vi "Generate intial guess.vi"(2 "数组":dbl[][](array[numeric])) -> (14 "peak":dbl, 15 "xc":dbl, 16 "yc":dbl, 17 "sigx":i32, 18 "sigy":i32)   [LabVIEW 2013]
panel:
  out "数组 3":ext[](array[numeric])
  out "数组 2":dbl[](array[numeric])
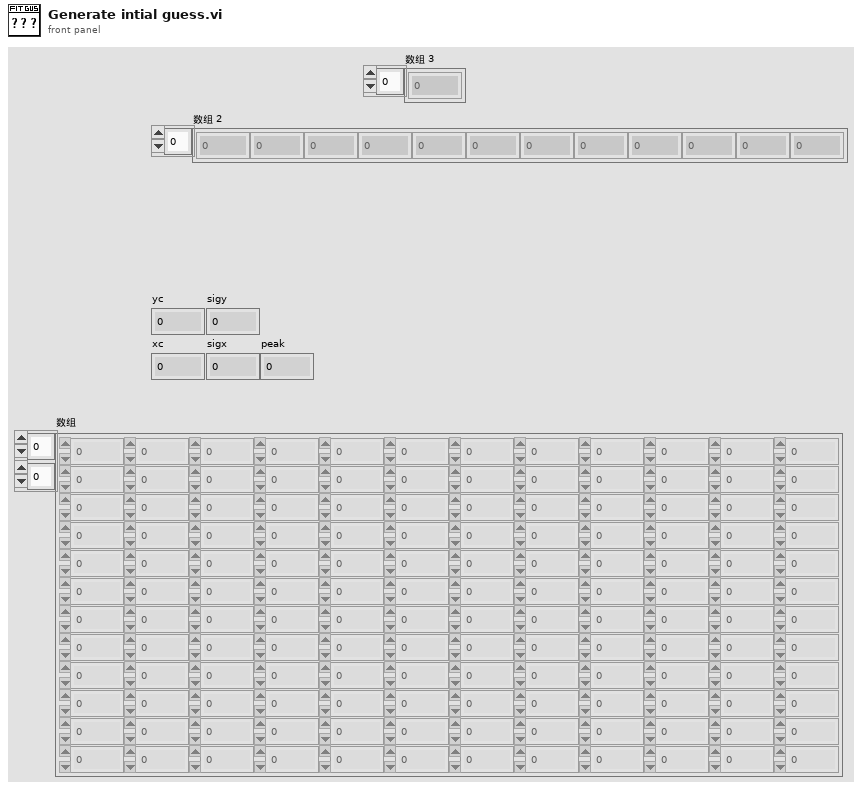
[diagram p1: front panel]
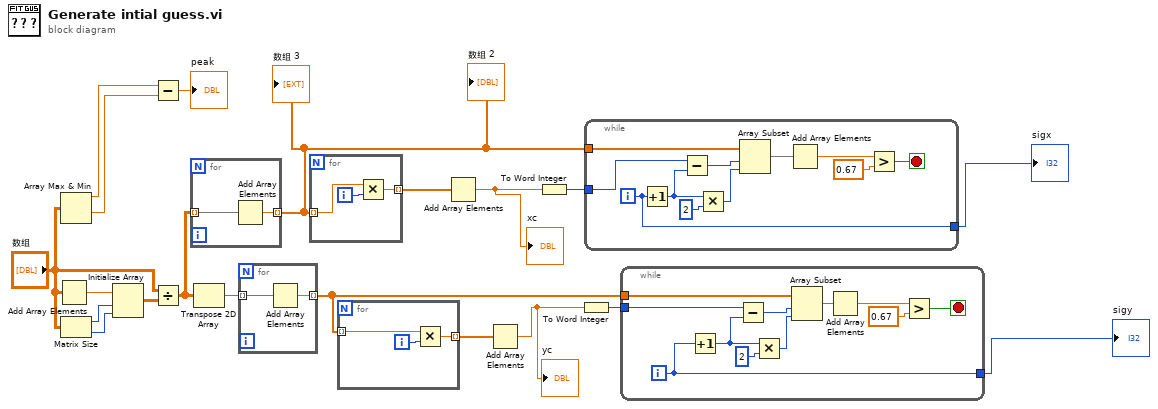
[diagram p0: block diagram]
diagram:
  n1 = Add Array Elements(numeric array="数组") -> (sum=w18:dbl)
  n2 = Array Max & Min(array="数组") -> (max value=w7:dbl, min value=w6:dbl)  [unwired: 2 out]
  n3 = Matrix Size(0:"数组") -> (1:w20:i32, 2:w19:i32)
  n4 = Initialize Array(w18, w20, w19) -> (w17:dbl[][])
  n5 = Subtract(x=w7, y=w6) -> (x-y=→"peak":dbl)
  n6 = Divide(x="数组", y=w17) -> (x/y=w16:dbl[][])
  n7 = for {
    tunnel: w16 -> [w22] mode=indexing
    tunnel: [w21] -> w10 mode=indexing
    n8 = Add Array Elements(numeric array=w22) -> (sum=w21:dbl)
  }
  "数组 2" <- w10
  "数组 3" <- w10
  n9 = Transpose 2D Array(2D array=w16) -> (transposed array=w15:dbl[][])
  n10 = for {
    tunnel: w15 -> [w24] mode=indexing
    tunnel: [w23] -> w11 mode=indexing
    n11 = Add Array Elements(numeric array=w24) -> (sum=w23:dbl)
  }
  n12 = for {
    tunnel: w10 -> [w26] mode=indexing
    tunnel: [w25] -> w13 mode=indexing
    i -> [w27]
    n13 = Multiply(x=w26, y=w27) -> (x*y=w25:dbl)
  }
  n14 = for {
    tunnel: w11 -> [w29] mode=indexing
    tunnel: [w28] -> w14 mode=indexing
    i -> [w30]
    n15 = Multiply(x=w29, y=w30) -> (x*y=w28:dbl)
  }
  n16 = Add Array Elements(numeric array=w13) -> (sum=w4:dbl)
  "xc" <- w4
  n17 = Add Array Elements(numeric array=w14) -> (sum=w3:dbl)
  "yc" <- w3
  n18 = To Word Integer(number=w4) -> (16bit integer=w9:i16)
  n19 = To Word Integer(number=w3) -> (16bit integer=w12:i16)
  n20 = while {
    tunnel: w9 -> [w41]
    tunnel: w10 -> [w36]
    tunnel: [w31] -> w2
    i -> [w31]
    stop <- w32 stop-if-true
    n21 = Increment(x=w31) -> (x+1=w39:i32)
    n22 = Subtract(x=w41, y=w39) -> (x-y=w40:i32)
    n23 = Multiply(x=w39, y=2) -> (x*y=w37:i32)
    n24 = Array Subset(array=w36, index=w40, length=w37) -> (w35:dbl[])
    n25 = Add Array Elements(numeric array=w35) -> (sum=w34:dbl)
    n26 = Greater?(x=w34, y=0.67) -> (0:w32:bool)
  }
  "sigx" <- w2
  n27 = while {
    tunnel: w12 -> [w52]
    tunnel: w11 -> [w47]
    tunnel: [w42] -> w1
    i -> [w42]
    stop <- w43 stop-if-true
    n28 = Increment(x=w42) -> (x+1=w50:i32)
    n29 = Subtract(x=w52, y=w50) -> (x-y=w51:i32)
    n30 = Multiply(x=w50, y=2) -> (x*y=w48:i32)
    n31 = Array Subset(array=w47, index=w51, length=w48) -> (w46:dbl[])
    n32 = Add Array Elements(numeric array=w46) -> (sum=w45:dbl)
    n33 = Greater?(x=w45, y=0.67) -> (0:w43:bool)
  }
  "sigy" <- w1
